vi "VelToTics.vi"(11 "Velocity/Sec":i16) -> (2 "Periods/tic":fxp<+,32,0> format="%.32g", 3 "Direction":bool)   [LabVIEW 2015]
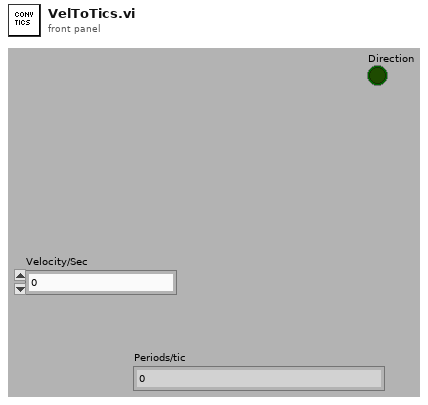
[diagram p1: front panel]
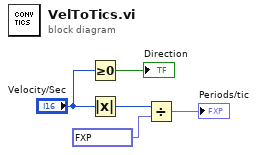
[diagram p0: block diagram]
diagram:
  n1 = Greater Or Equal To 0?(x="Velocity/Sec") -> (x >= 0?=→"Direction":bool)
  n2 = Absolute Value(x="Velocity/Sec") -> (abs(x)=w3:i16)
  n3 = Divide(x=w3, y=fxp<+,17,28> 160000000.0) -> (x/y=→"Periods/tic":fxp<+,32,0>)
